vi "Read Position_Tiles.vi"(8 "error in (no error)":errorcluster, 11 "BounceTarget in":refnum<class "BounceTarget.lvclass">) -> (0 "error out":errorcluster, 2 "Coordinate":T1, 3 "BounceTarget out":refnum<class "BounceTarget.lvclass">)   [LabVIEW 2019, in "RT_Game.lvlib" / "BounceTarget.lvclass"]
uses:
  BounceTarget.lvclass
  Engine/Coordinate.ctl
  BounceTarget.lvclass/BounceTarget.ctl
  Engine/Engine.lvclass
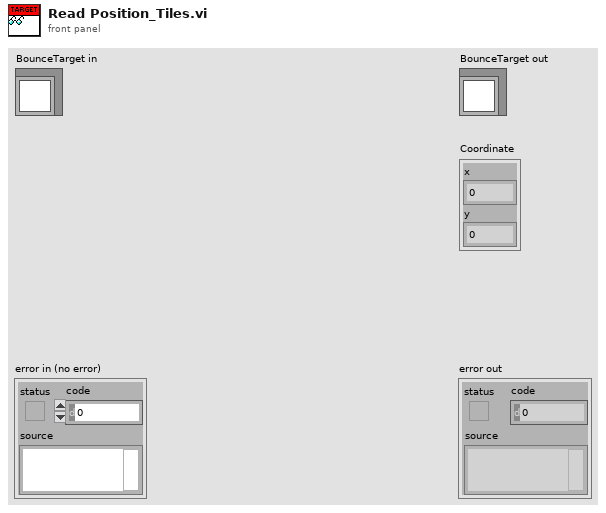
[diagram p1: front panel]
types:
  T1 = typedef "RT_Game.lvlib/Engine.lvclass/Coordinate.ctl" = cluster{"x":dbl, "y":dbl}
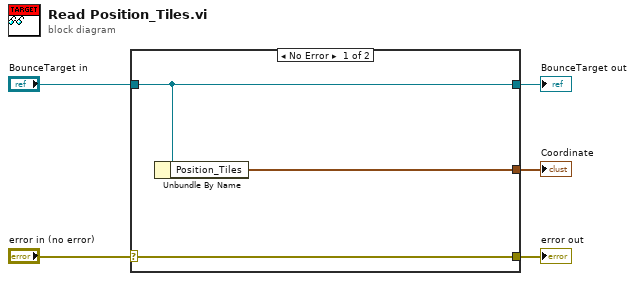
[diagram p0: block diagram]
diagram:
  n1 = case shown="No Error" "error in (no error)" {
    selector: "error in (no error)" -> [w8 w9]
    tunnel: [w8 w9] -> w4
    tunnel: [w7 w10] -> w2
    tunnel: "BounceTarget in" -> [w7 w10]
    tunnel: [w6 _] -> w1
    frame No Error {
      n2 = Unbundle By Name(w7) -> ("Position_Tiles"=w6:T1)
    }
    frame Error {
    }
  }
  "error out" <- w4
  "BounceTarget out" <- w2
  "Coordinate" <- w1
